vi "PointerArray_Get Pointer.vi"(6 "Create If Not Found":bool=TRUE, 8 "Error":errorcluster, 9 "Pointer":refnum<class "((Pointer)).lvclass">, 10 "Index":i32=-1, 11 "Pointer Array":refnum<class "((Pointer)).lvclass">[](array[class])) -> (0 "Error Out":errorcluster, 1 "Pointer Out":refnum<class "((Pointer)).lvclass">, 2 "Index Out":i32, 3 "Pointer Array Out":refnum<class "((Pointer)).lvclass">[](array[class]), 4 "Found Out":bool)   [LabVIEW 2016, in "(WavBuf).lvclass"]
uses:
  (WavBuf).lvclass
  Pointer/((Pointer)).lvclass
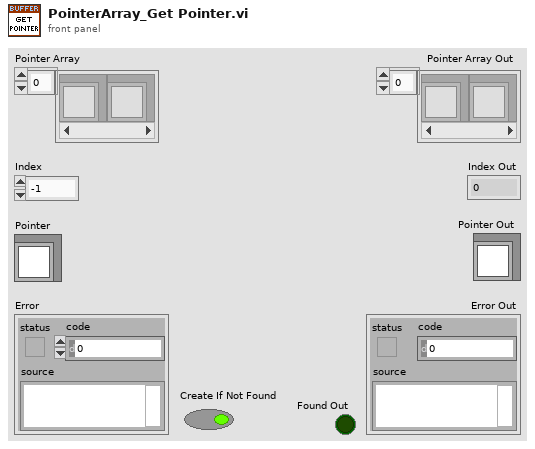
[diagram p1: front panel]
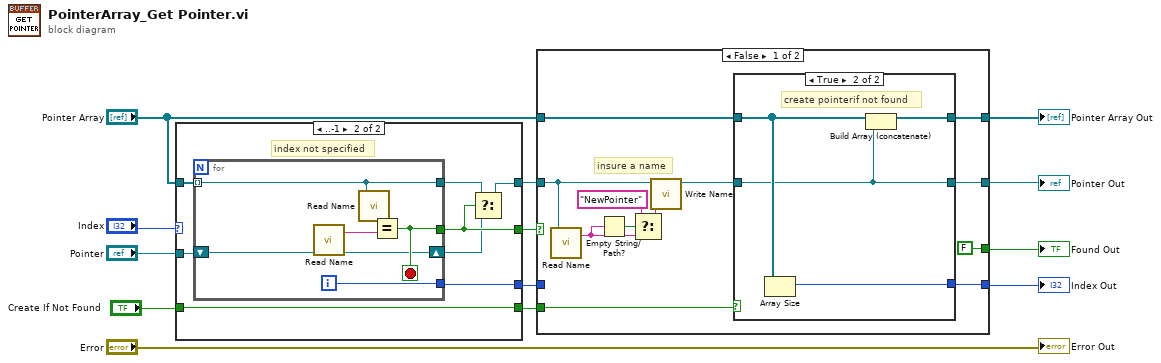
[diagram p0: block diagram]
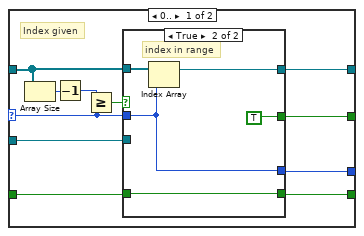
[diagram p2: hidden frame]
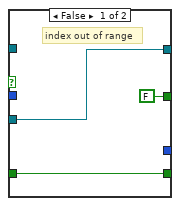
[diagram p3: hidden frame]
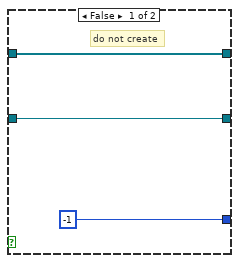
[diagram p4: hidden frame]
diagram:
  n1 = case shown="..-1" "Index" {
    selector: "Index" -> [w20 _]
    tunnel: "Pointer" -> [w14 w40]
    tunnel: [w17 w36] -> w11
    tunnel: "Pointer Array" -> [w23 w39]
    tunnel: [w19 w33] -> w9
    tunnel: [w18 w38] -> w8
    tunnel: [w16 w37] -> w4
    tunnel: "Create If Not Found" -> [w15 w37]
    frame 0.. {
      # "Index given"
      n2 = Array Size(array=w23) -> (size(s)=w24:i32)
      n3 = Decrement(x=w24) -> (x-1=w22:i32)
      n4 = Greater Or Equal?(x=w22, y=w20) -> (x >= y?=w21:bool)
      n5 = case shown="True" w21 {
        tunnel: w23 -> [_ w32]
        tunnel: w20 -> [_ w31]
        tunnel: [w25 w28] -> w19
        tunnel: [_ w31] -> w18
        tunnel: [FALSE TRUE] -> w17
        tunnel: [w26 w29] -> w16
        tunnel: w15 -> [w26 w29]
        tunnel: w14 -> [w25 _]
        frame False {
          # "index out of range"
        }
        frame True {
          # "index in range"
          n6 = Index Array(array=w32, index=w31) -> (element=w28:refnum<class "((Pointer)).lvclass">)
        }
      }
    }
    frame ..-1 {
      # "index not specified"
      n7 = for {
        tunnel: w39 -> [w43] mode=indexing
        tunnel: [w43] -> w34
        tunnel: [w45] -> w36
        tunnel: [w44] -> w38
        shift-right: [w42] -> w35
        shift-left: w40 -> [w42]
        i -> [w44]
        stop <- w45 stop-if-true
        n8 = call "Read Name.vi"("((Pointer))"=w42) -> ("Name Out"=w41:string)  [unwired: 2 in]
        n9 = call "Read Name.vi"("((Pointer))"=w43) -> ("Name Out"=w46:string)  [unwired: 2 in]
        n10 = Equal?(x=w46, y=w41) -> (x = y?=w45:bool)
      }
      n11 = Select(t=w34, s=w36, f=w35) -> (s? t:f=w33:refnum<class "((Pointer)).lvclass">)
    }
  }
  n12 = case shown="False" w11 {
    selector: w11 -> [_ w67]
    tunnel: "Pointer Array" -> [w56 w69]
    tunnel: w9 -> [w47 w66]
    tunnel: w8 -> [_ w68]
    tunnel: [w57 w68] -> w7
    tunnel: [FALSE w67] -> w6
    tunnel: [w55 w69] -> w5
    tunnel: w4 -> [w54 _]
    tunnel: [w48 w66] -> w1
    frame False {
      # "insure a name"
      n13 = call "Read Name.vi"("((Pointer))"=w47) -> ("Name Out"=w51:string)  [unwired: 2 in]
      n14 = Empty String/Path?(string/path=w51) -> (empty?=w53:bool)
      n15 = Select(t="NewPointer" ("Name"), s=w53, f=w51) -> (s? t:f=w50:string)
      n16 = call-dynamic "Write Name.vi"("Name"=w50, "((Pointer)) in"=w47) -> ("((Pointer)) out"=w49:refnum<class "((Pointer)).lvclass">)  [unwired: 9 in]
      n17 = case shown="True" w54 {
        tunnel: w49 -> [w59 w62]
        tunnel: [-1 w65] -> w57
        tunnel: [w59 w62] -> w48
        tunnel: w56 -> [w61 w64]
        tunnel: [w61 w63] -> w55
        frame False {
          # "do not create"
        }
        frame True {
          # "create pointerif not found"
          n18 = Array Size(array=w64) -> (size(s)=w65:i32)
          n19 = Build Array (concatenate)(w64, w62) -> (w63:refnum<class "((Pointer)).lvclass">[])
        }
      }
    }
    frame True {
    }
  }
  "Pointer Out" <- w1
  "Pointer Array Out" <- w5
  "Index Out" <- w7
  "Found Out" <- w6
  "Error Out" <- "Error"
